vi "Unflatten.vi"(8 "error in (no error)":errorcluster, 11 "Continuous in":refnum<class "Continuous.lvclass">) -> (0 "error out":errorcluster, 3 "Continuous out":refnum<class "Continuous.lvclass">)   [LabVIEW 2009, in "Continuous.lvclass"]
uses:
  Continuous.lvclass
  Scanner/Scanner.lvclass
  Global/File Locations.vi
  Continuous.lvclass/Continuous.ctl
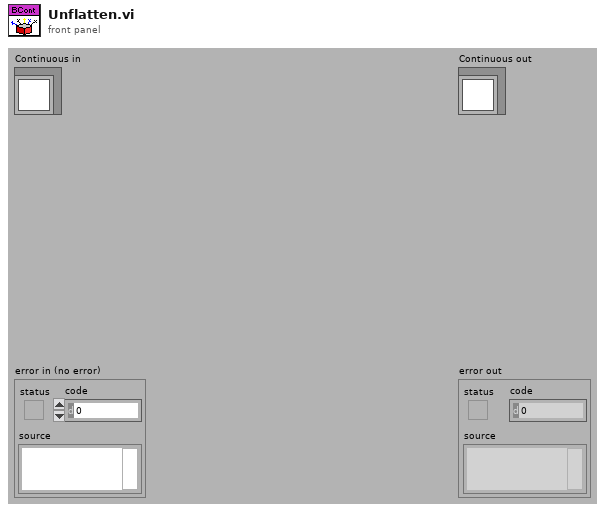
[diagram p1: front panel]
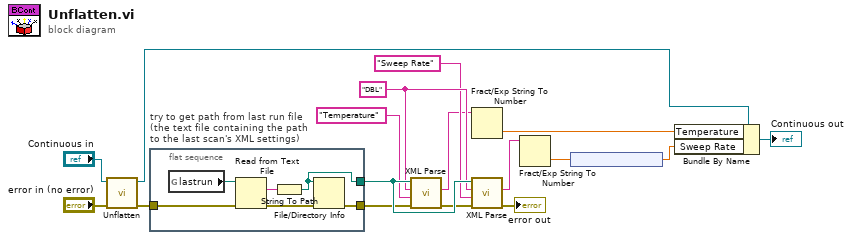
[diagram p0: block diagram]
diagram:
  w11 = "DBL"
  n1 = call-parent "Unflatten.vi"("error in (no error)"="error in (no error)", "Scanner in"="Continuous in") -> ("error out"=w14:errorcluster, "Scanner out"=w17:refnum<class "Continuous.lvclass">)  [unwired: 8 in]
  n2 = flat-sequence "try to get path from last run file\n(the text file containing the path\nto the last scan's XML settings)" {
    tunnel: [w23] -> w12
    tunnel: [w19] -> w8
    tunnel: w14 -> [w18]
    frame #0 {
      n3 = global read "File Locations.vi" "lastrun"() -> (w21:path)
      n4 = Read from Text File(file (use dialog)=w21, error in=w18) -> (text=w22:string, error out=w20:errorcluster)  [unwired: 4 out]
      n5 = String To Path(string=w22) -> (path=w23:path)
      n6 = File/Directory Info(path=w23, error in=w20) -> (error out=w19:errorcluster)  [unwired: 6 out]
    }
  }
  n7 = call "XML Parse.vi"("error in (no error)"=w8, "Name String"="Temperature", "Type String"=w11, "Path"=w12) -> ("error out"=w7:errorcluster, "String Out"=w5:string)  [unwired: 6 in]
  n8 = Fract/Exp String To Number(string=w5) -> (number=w2:dbl)  [unwired: 3 in, 1 out]
  n9 = call "XML Parse.vi"("error in (no error)"=w7, "Name String"="Sweep Rate", "Type String"=w11, "Path"=w12) -> ("error out"=→"error out":errorcluster, "String Out"=w4:string)  [unwired: 6 in]
  n10 = Fract/Exp String To Number(string=w4) -> (number=w3:dbl)  [unwired: 3 in, 1 out]
  n11 = node(w3) -> (w1:dbl[unit])
  n12 = Bundle By Name(cluster=w17, "Temperature"=w2, "Sweep Rate"=w1) -> (→"Continuous out":refnum<class "Continuous.lvclass">)
